vi "Send CameraOpticsDiagnosticsResult_SM.vi"(7 "Message Priority (Normal)":T3=enum."Normal", 8 "error in (no error)":errorcluster, 10 "Camera Optics Diagnostics Result":T1={"LightCameraName"="", "DiagnosedImage"=refnum, "DustPercentage"=0.0, "Result"=TRUE}, 11 "Message Enqueuer":refnum<class "Message Enqueuer.lvclass">) -> (0 "error out":errorcluster, 3 "Message Enqueuer out":refnum<class "Message Enqueuer.lvclass">)   [LabVIEW 2019, in "CameraOpticsDiagnosticsResult_SM Msg.lvclass"]
doc: "This VI sends the message to an actor."
uses:
  CameraOpticsDiagnosticsResult_SM Msg.lvclass
  <vilib>/ActorFramework/Message Enqueuer/Message Enqueuer.lvclass
  C:/Program Files/National Instruments/LabVIEW 2019/vi.lib/ActorFramework/Message/Message.lvclass
  <vilib>/ActorFramework/Message Enqueuer/Message Priority.ctl
  <vilib>/vision/Image Controls.llb/IMAQ Image.ctl
  Common/Controls/Camera Optics Diagnostics Result.ctl
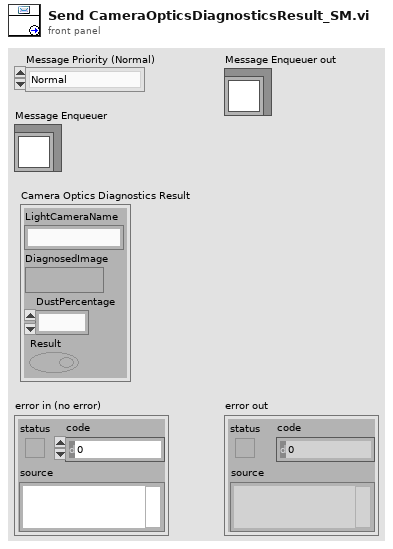
[diagram p1: front panel]
types:
  T1 = typedef "Camera Optics Diagnostics Result.ctl" = cluster{"LightCameraName":string, "DiagnosedImage":T2, "DustPercentage":dbl, "Result":bool}
  T2 = typedef "IMAQ Image.ctl" = refnum<image>
  T3 = typedef "Actor Framework.lvlib/Message Enqueuer.lvclass/Message Priority.ctl" = enum16{"Low", "Normal", "High"}
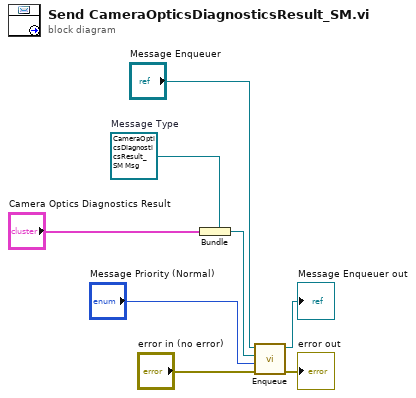
[diagram p0: block diagram]
diagram:
  w5 = refnum<class "CameraOpticsDiagnosticsResult_SM Msg.lvclass"> refnum  # Message Type
  n1 = Bundle(cluster=w5, "Camera Optics Diagnostics Result") -> (w4:refnum<class "CameraOpticsDiagnosticsResult_SM Msg.lvclass">)
  n2 = call <vilib>:"Enqueue.vi"("error in (no error)"="error in (no error)", "Message Priority (Normal)"="Message Priority (Normal)", "Message"=w4, "Message Enqueuer in"="Message Enqueuer") -> ("error out"=→"error out":errorcluster, "Message Enqueuer out"=→"Message Enqueuer out":refnum<class "Message Enqueuer.lvclass">)  [unwired: 6 in]
